vi "OPEN & CONFIG INTAKE.vi"(0 "INTAKE DRIVE refname":string="INTAKE DRIVE", 1 "INTAKE DRIVE CAN ID":u8=8, 3 "INTAKE LIFT refname":string="INTAKE LIFT", 4 "INTAKE LIFT CAN ID":u8=4, 9 "LIFT PID Constants":T1={"P Gain"=1.0, "I Gain"=0.0, "D Gain"=0.0, "F Gain"=0.0, "I Zone"=0.0, "Min Output"=-0.5, "Max Output"=0.5} {"Max Output" min=-1.0 max=1.0 step=0.01; "Min Output" min=-1.0 max=1.0 step=0.01; "I Zone" step=0.01; "F Gain" step=0.01; "D Gain" step=0.01; "I Gain" step=0.01; "P Gain" min=0.0 step=0.01}) -> ()   [LabVIEW 2020]
uses:
  <vilib>/Rock Robotics/WPI/ThirdParty/REV Robotics/REVLib/Typedef/Spark MAX Idle Mode.ctl
  <vilib>/Rock Robotics/WPI/ThirdParty/REV Robotics/REVLib/Typedef/Spark MAX Motor Type.ctl
  <vilib>/Rock Robotics/WPI/ThirdParty/REV Robotics/REVLib/Typedef/Spark MAX Limit Direction.ctl
  <vilib>/Rock Robotics/WPI/ThirdParty/Phoenix-LabVIEW/Motor Controller/Controls/CTRE_Phoenix_MotorControl_NeutralMode.ctl
  <vilib>/Rock Robotics/WPI/ThirdParty/Phoenix-LabVIEW/Motor Controller/Controls/CTRE_Phoenix_MotorControl_TalonFXInvertType.ctl
  <vilib>/Rock Robotics/Network Tables/NT Write Boolean.vi
panel:
  out "motor revs":dbl=9.0
  in  "deploy angle (deg)":dbl=135.0
  in  "sprocket teeth on motor":dbl=16.0
  in  "sprocket teeth on shaft":dbl=32.0
  in  "PLANETARY GEAR ratio":dbl=12.0
  in  "Idle Mode LIFT":T2=enum."Brake"
  in  "Idle Mode DRIVE":T2
  in  "Invert INTAKE LIFT?":bool
  in  "Invert INTAKE DRIVE?":bool=TRUE
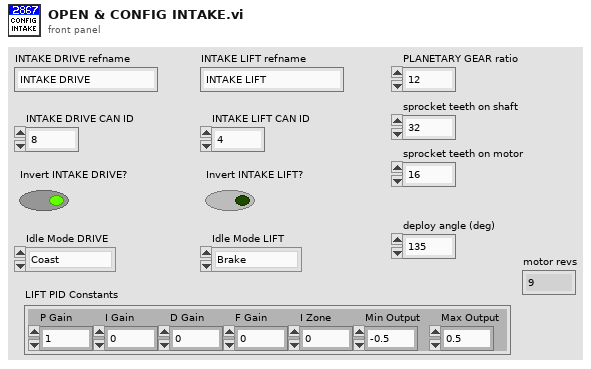
[diagram p1: front panel]
types:
  T1 = cluster{"P Gain":dbl, "I Gain":dbl, "D Gain":dbl, "F Gain":dbl, "I Zone":dbl, "Min Output":dbl, "Max Output":dbl}
  T2 = typedef "Spark MAX Idle Mode.ctl" = enum16{"Coast", "Brake"}
  T3 = typedef "CTRE_Phoenix_MotorControl_NeutralMode.ctl" = enum8{"EEPROMSetting", "Override to Coast", "Override to Brake"}
  T4 = typedef "CTRE_Phoenix_MotorControl_TalonFXInvertType.ctl" = enum16{"Counter-Clockwise", "Clockwise"}
  T5 = typedef "WPI_MotorControlDeviceRef.ctl" = cluster{"DeviceStatus":errorcluster, "Type":T6, "PWM":cluster{"PWM Channel":T7, "DeadBand":T8}, "CAN":cluster{"Device Number":u8, "SetOutput VI Ref":variant, "GetOutput VI Ref":variant, "Enable VI Ref":variant, "Disable VI Ref":variant, "Data":variant}, "Invert":bool, "DIO PWM":cluster{"PWM \"Enable\" Channel":T7, "DIOChannel":T9, "PWM Rate":dbl}}
  T6 = typedef "WPI_MotorControlType.ctl" = enum16{"PWM", "CAN", "DIO PWM"}
  T7 = typedef "FPGA_DIOPWMChannel.ctl" = enum8{"PWM 0", "PWM 1", "PWM 2", "PWM 3", "PWM 4", "PWM 5", "PWM 6", "PWM 7", "PWM 8", "PWM 9", "PWM MXP 0", "PWM MXP 1", "PWM MXP 2", "PWM MXP 3", "PWM MXP 4", "PWM MXP 5", "PWM MXP 6", "PWM MXP 7", "PWM MXP 8", "PWM MXP 9", "Invalid"}
  T8 = typedef "WPI_PWMDeadband.ctl" = cluster{"Name":string, "maxPositivePwm":i32, "minPositivePwm":i32, "centerPwm":i32, "maxNegativePwm":i32, "minNegativePwm":i32, "angularRange":u16}
  T9 = typedef "FPGA_DIOChannel.ctl" = enum8{"DIO 0", "DIO 1", "DIO 2", "DIO 3", "DIO 4", "DIO 5", "DIO 6", "DIO 7", "DIO 8", "DIO 9", "DIO MXP 0", "DIO MXP 1", "DIO MXP 2", "DIO MXP 3", "DIO MXP 4", "DIO MXP 5", "DIO MXP 6", "DIO MXP 7", "DIO MXP 8", "DIO MXP 9", "DIO MXP 10", "DIO MXP 11", "DIO MXP 12", "DIO MXP 13", "DIO MXP 14", "DIO MXP 15", "SPI Port CS1", "SPI Port CS2", "SPI Port CS3", "SPI Port MISO", "SPI Port MOSI", "Invalid"}
  T10 = typedef "Spark MAX Limit Direction.ctl" = enum16{"Forward Limit", "Reverse Limit"}
  T11 = typedef "Spark MAX Motor Type.ctl" = enum16{"Brushed", "Brushless"}
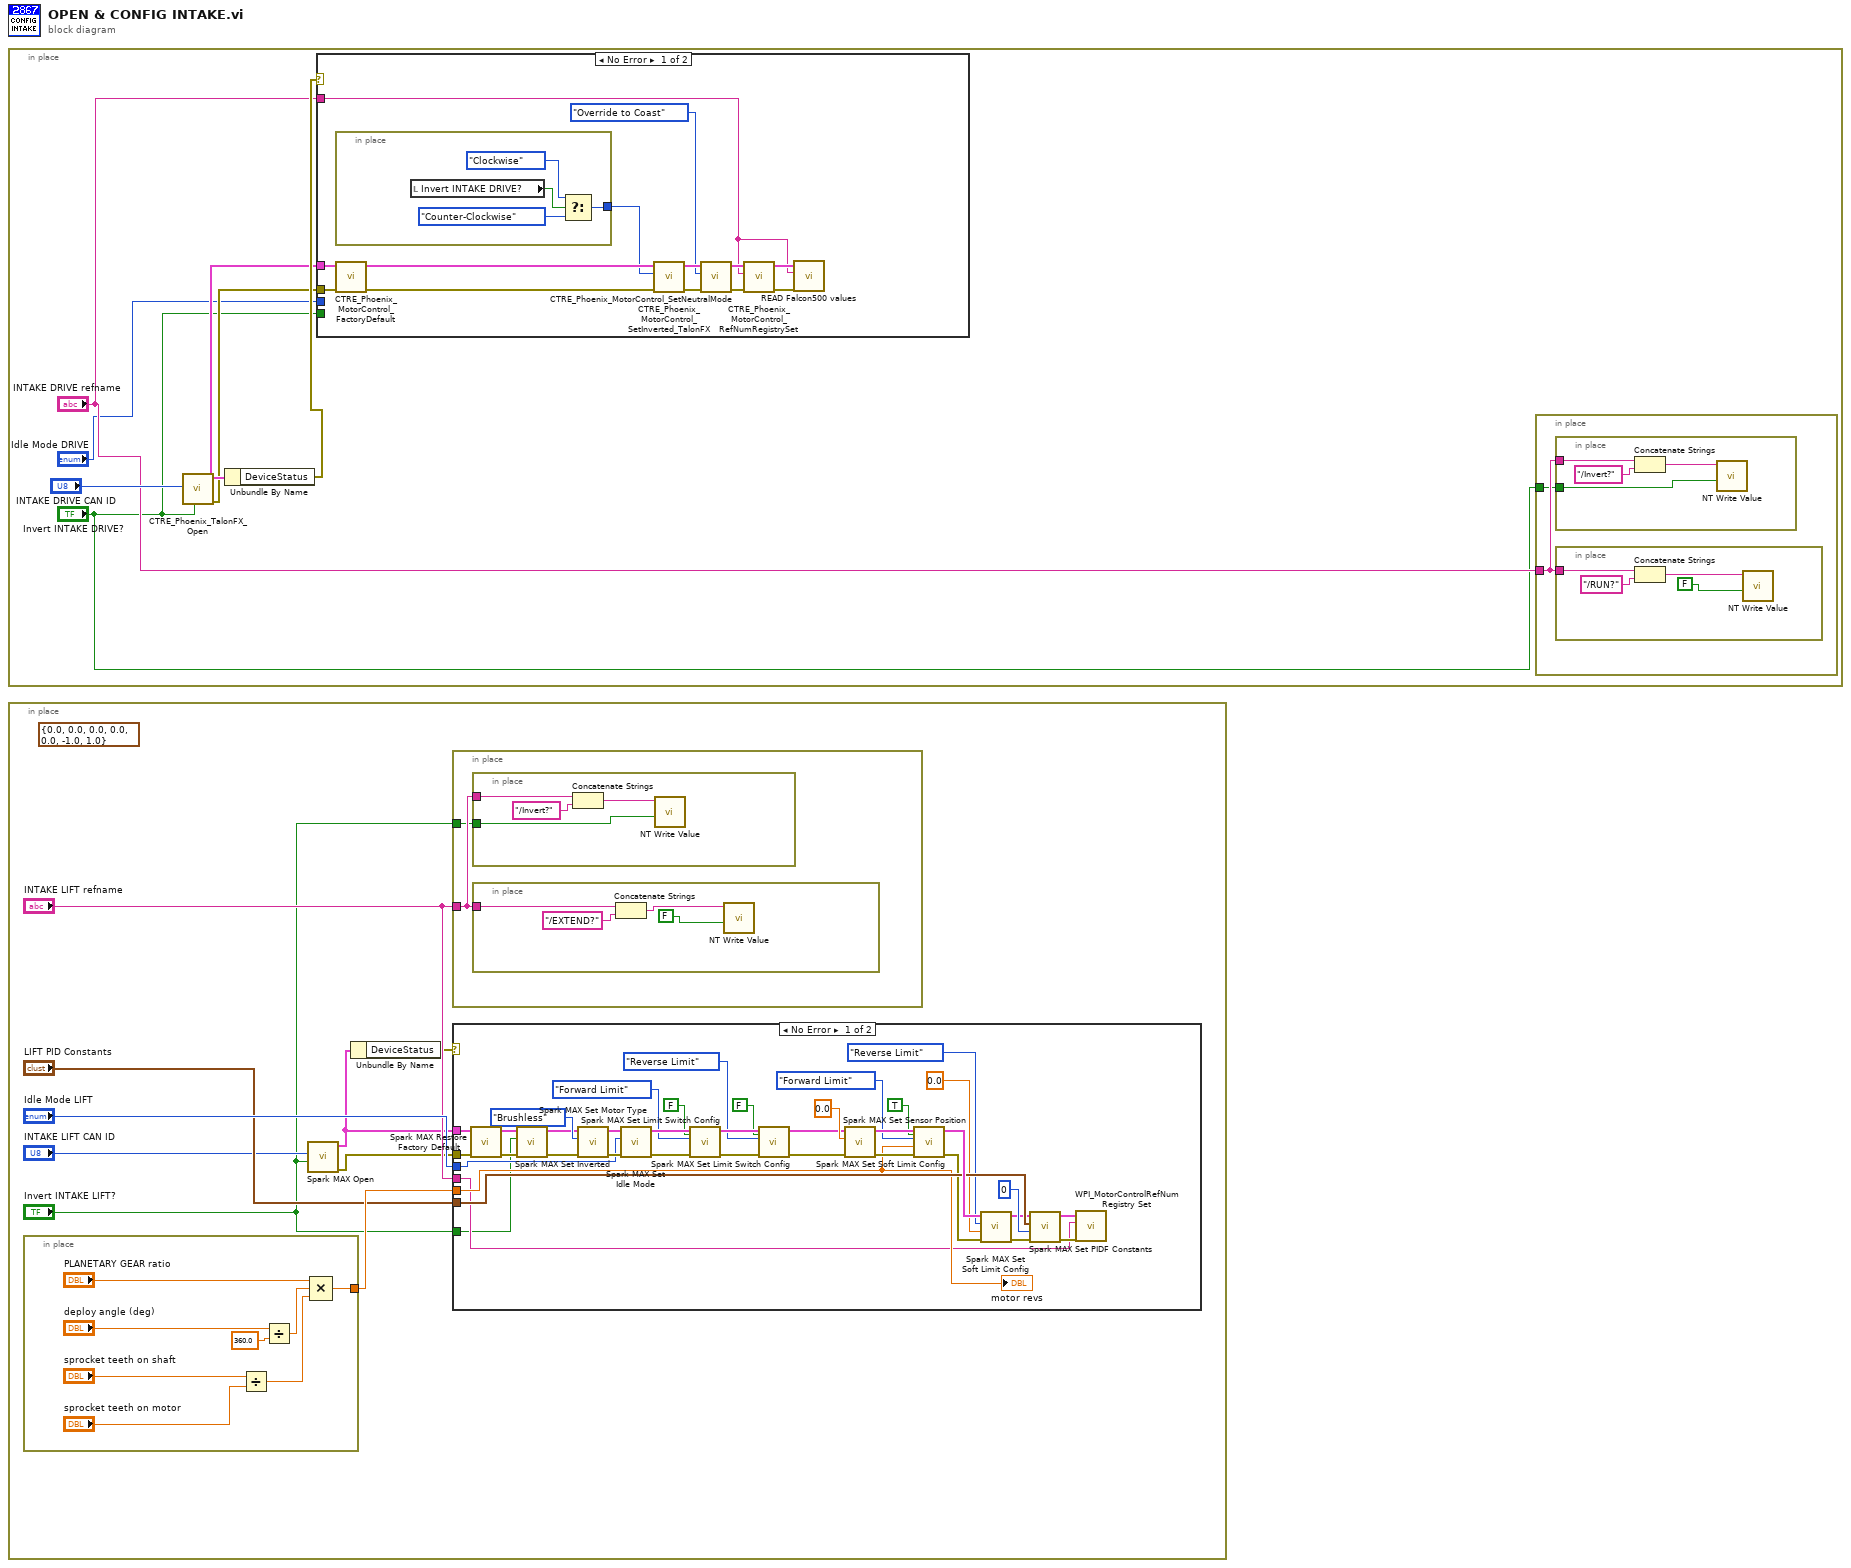
[diagram p0: block diagram]
diagram:
  n1 = in-place {
    n2 = call <vilib>:"CTRE_Phoenix_TalonFX_Open.vi"("Invert"="Invert INTAKE DRIVE?", "Device Number"="INTAKE DRIVE CAN ID") -> ("error out"=w4:errorcluster, "PhoenixMotorControlDevRef"=w5:T5)  [unwired: 8 in]
    n3 = Unbundle By Name(w5) -> ("DeviceStatus"=w6:errorcluster)
    n4 = case shown="No Error" w6 {
      tunnel: w5 -> [w20 _]
      tunnel: w4 -> [w19 _]
      tunnel: "INTAKE DRIVE refname" -> [w8 _]
      tunnel: "Idle Mode DRIVE" -> [_ _]
      tunnel: "Invert INTAKE DRIVE?" -> [_ _]
      frame No Error {
        n5 = in-place {
          in-place-border: [w22] -> w16
          n6 = local read "Invert INTAKE DRIVE?"() -> (w21:bool)
          n7 = Select(t=CTRE_Phoenix_MotorControl_TalonFXInvertType."Clockwise" ("Invert Type"), s=w21, f=CTRE_Phoenix_MotorControl_TalonFXInvertType."Counter-Clockwise" ("Invert Type")) -> (s? t:f=w22:T4)
        }
        n8 = call <vilib>:"CTRE_Phoenix_MotorControl_FactoryDefault.vi"("error in"=w19, "PhoenixMotorControlDevRef"=w20) -> ("error out"=w18:errorcluster, "PhoenixMotorControlDevRef"=w17:T5)  [unwired: 8 in]
        n9 = call <vilib>:"CTRE_Phoenix_MotorControl_SetInverted_TalonFX.vi"("error in (no error)"=w18, "Invert Type"=w16, "PhoenixMotorControlDevRef"=w17) -> ("error out"=w15:errorcluster, "PhoenixMotorControlDevRef"=w14:T5)  [unwired: 7 in]
        n10 = call <vilib>:"CTRE_Phoenix_MotorControl_SetNeutralMode.vi"("error in (no error)"=w15, "Motor Control Neutral Mode"=CTRE_Phoenix_MotorControl_NeutralMode."Override to Coast", "PhoenixMotorControlDevRef"=w14) -> ("error out"=w12:errorcluster, "PhoenixMotorControlDevRef"=w11:T5)  [unwired: 7 in]
        n11 = call <vilib>:"CTRE_Phoenix_MotorControl_RefNumRegistrySet.vi"("error in (no error)"=w12, "refnum name"=w8, "PhoenixMotorControlDevRef"=w11) -> ("error out"=w9:errorcluster, "PhoenixMotorControlDevRef"=w10:T5)  [unwired: 7 in]
        n12 = call "READ Falcon500 values.vi"("PhoenixMotorControlDevRef"=w10, "refnum name"=w8, "error in (no error)"=w9) -> ()  [unwired: 5 in, 2 out]
      }
      frame Error {
      }
    }
    n13 = in-place {
      in-place-border: "INTAKE DRIVE refname" -> [w26]
      in-place-border: "Invert INTAKE DRIVE?" -> [w25]
      n14 = in-place {
        in-place-border: w26 -> [w28]
        in-place-border: w25 -> [w27]
        n15 = Concatenate Strings(w28, "/Invert?" ("string")) -> (w30:string)
        n16 = call-poly <vilib>:"NT Write Value.vi"("Boolean"=w27, "Name"=w30) -> ()  [unwired: 9 in, 1 out]
      }
      n17 = in-place {
        in-place-border: w26 -> [w31]
        n18 = Concatenate Strings(w31, "/RUN?" ("string")) -> (w34:string)
        n19 = call-poly <vilib>:"NT Write Value.vi"("Boolean"=FALSE, "Name"=w34) -> ()  [unwired: 9 in, 1 out]
      }
    }
  }
  n20 = in-place {
    (unwired) T1 {"P Gain"=0.0, "I Gain"=0.0, "D Gain"=0.0, "F Gain"=0.0, "I Zone"=0.0, "Min Output"=-1.0, "Max Output"=1.0} ("PID Constants")
    n21 = in-place {
      in-place-border: [w92] -> w42
      n22 = Divide(x="sprocket teeth on shaft", y="sprocket teeth on motor") -> (x/y=w97:dbl)
      n23 = Divide(x="deploy angle (deg)", y=360.0) -> (x/y=w96:dbl)
      n24 = Compound Arithmetic op=MULTIPLY("PLANETARY GEAR ratio", w96, w97) -> (w92:dbl)
    }
    n25 = call <vilib>:"Spark MAX Open.vi"("Invert"="Invert INTAKE LIFT?", "Device Number"="INTAKE LIFT CAN ID") -> ("error out"=w39:errorcluster, "MotorControlDeviceRef"=w37:T5)  [unwired: 8 in]
    n26 = Unbundle By Name(w37) -> ("DeviceStatus"=w38:errorcluster)
    n27 = in-place {
      in-place-border: "INTAKE LIFT refname" -> [w83]
      in-place-border: "Invert INTAKE LIFT?" -> [w82]
      n28 = in-place {
        in-place-border: w83 -> [w85]
        in-place-border: w82 -> [w84]
        n29 = Concatenate Strings(w85, "/Invert?" ("string")) -> (w87:string)
        n30 = call-poly <vilib>:"NT Write Value.vi"("Boolean"=w84, "Name"=w87) -> ()  [unwired: 9 in, 1 out]
      }
      n31 = in-place {
        in-place-border: w83 -> [w88]
        n32 = Concatenate Strings(w88, "/EXTEND?" ("string")) -> (w91:string)
        n33 = call-poly <vilib>:"NT Write Value.vi"("Boolean"=FALSE, "Name"=w91) -> ()  [unwired: 9 in, 1 out]
      }
    }
    n34 = case shown="No Error" w38 {
      tunnel: w37 -> [w81 _]
      tunnel: "Idle Mode LIFT" -> [w69 _]
      tunnel: w42 -> [w60 _]
      tunnel: "LIFT PID Constants" -> [w62 _]
      tunnel: "INTAKE LIFT refname" -> [w50 _]
      tunnel: w39 -> [w45 _]
      tunnel: "Invert INTAKE LIFT?" -> [w44 _]
      frame No Error {
        n35 = call <vilib>:"Spark MAX Restore Factory Default.vi"("error in"=w45, "MotorControlDeviceRef"=w81) -> ("error out"=w46:errorcluster, "MotorControlDeviceRef"=w49:T5)  [unwired: 8 in]
        n36 = call <vilib>:"Spark MAX Set Inverted.vi"("error in (no error)"=w46, "Inverted (F)"=w44, "MotorControlDeviceRef in"=w49) -> ("error out"=w47:errorcluster, "MotorControlDeviceRef out"=w48:T5)  [unwired: 7 in]
        n37 = call <vilib>:"Spark MAX Set Motor Type.vi"("error in (no error)"=w47, "Motor Type"=Spark_MAX_Motor_Type."Brushless", "MotorControlDevRef"=w48) -> ("error out"=w79:errorcluster, "MotorControlDeviceRef"=w78:T5)  [unwired: 7 in]
        n38 = call <vilib>:"Spark MAX Set Idle Mode.vi"("error in (no error)"=w79, "Idle Mode"=w69, "MotorControlDeviceRef in"=w78) -> ("error out"=w77:errorcluster, "MotorControlDeviceRef out"=w76:T5)  [unwired: 7 in]
        n39 = call <vilib>:"Spark MAX Set Limit Switch Config.vi"("Enabled? (T)"=FALSE, "error in (no error)"=w77, "Limit Switch"=Spark_MAX_Limit_Direction."Forward Limit", "MotorControlDeviceRef in"=w76) -> ("error out"=w73:errorcluster, "MotorControlDeviceRef out"=w72:T5)  [unwired: 6 in]
        n40 = call <vilib>:"Spark MAX Set Limit Switch Config.vi"("Enabled? (T)"=FALSE, "error in (no error)"=w73, "Limit Switch"=Spark_MAX_Limit_Direction."Reverse Limit", "MotorControlDeviceRef in"=w72) -> ("error out"=w53:errorcluster, "MotorControlDeviceRef out"=w54:T5)  [unwired: 6 in]
        n41 = call <vilib>:"Spark MAX Set Sensor Position.vi"("error in"=w53, "Position"=0.0, "MotorControlDeviceRef"=w54) -> ("error out"=w67:errorcluster, "MotorControlDeviceRef"=w66:T5)  [unwired: 7 in]
        n42 = call <vilib>:"Spark MAX Set Soft Limit Config.vi"("Enabled? (T)"=TRUE, "error in (no error)"=w67, "Soft Limit (0)"=w60, "Soft Limit Switch"=Spark_MAX_Limit_Direction."Forward Limit", "MotorControlDeviceRef in"=w66) -> ("error out"=w58:errorcluster, "MotorControlDeviceRef out"=w63:T5)  [unwired: 5 in]
        n43 = call <vilib>:"Spark MAX Set Soft Limit Config.vi"("error in (no error)"=w58, "Soft Limit (0)"=0.0, "Soft Limit Switch"=Spark_MAX_Limit_Direction."Reverse Limit", "MotorControlDeviceRef in"=w63) -> ("error out"=w57:errorcluster, "MotorControlDeviceRef out"=w59:T5)  [unwired: 6 in]
        n44 = call <vilib>:"Spark MAX Set PIDF Constants.vi"("error in"=w57, "PIDF Slot"=0, "PID Constants"=w62, "MotorControlDeviceRef"=w59) -> ("error out"=w52:errorcluster, "MotorControlDeviceRef"=w51:T5)  [unwired: 6 in]
        n45 = call <vilib>:"WPI_MotorControlRefNum Registry Set.vi"("error in (no error)"=w52, "refnum name"=w50, "MotorControlDevRef"=w51) -> ()  [unwired: 7 in, 2 out]
        "motor revs" <- w60
      }
      frame Error {
      }
    }
  }
